vi "Wait On Timer Example 2.vi"() -> ()   [LabVIEW 2011]
panel:
  out "Exit":bool
  in  "Stop":bool
  out "Waveform Chart":dbl[](graph)
  in  "Time between chart updates (sec)":dbl=0.5 format="%.3f"
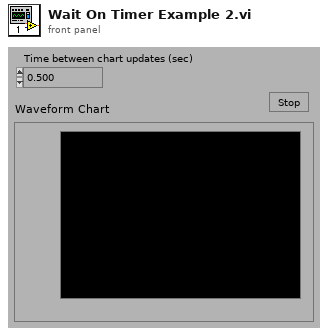
[diagram p1: front panel]
types:
  T1 = typedef "Timer Refnum.ctl" = refnum<k1>
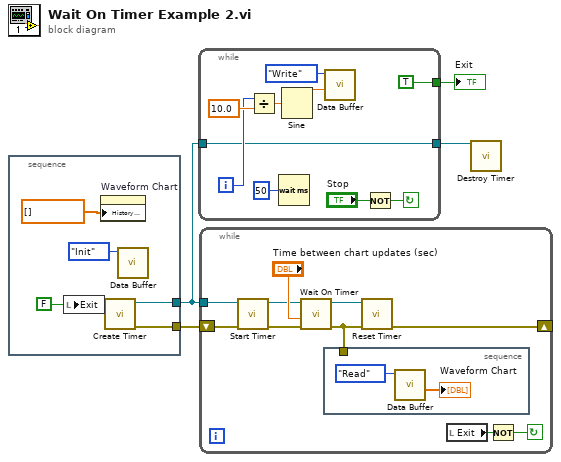
[diagram p0: block diagram]
diagram:
  n1 = stacked-sequence {
    tunnel: [w9] -> w3
    tunnel: [w8] -> w4
    frame #0 {
      n2 = local write "Exit"(FALSE ("Exit")) -> ()
      n3 = property on="Waveform Chart" class="WFChart (strict)"("History Data"=dbl[] [] ("Write Attribute")) -> ()  [unwired: 2 in, 2 out]
      n4 = call "Create Timer.vi"() -> ("error out"=w8:errorcluster, "timer"=w9:T1)  [unwired: 5 in, 1 out]
      n5 = call "Data Buffer.vi"("task"=enum16{"Init", "Write", "Read"}."Init") -> ()  [unwired: 6 in, 1 out]
    }
  }
  n6 = while {
    tunnel: [TRUE ("Stop")] -> w1
    tunnel: [w11] -> w2
    tunnel: w3 -> [w11]
    i -> [w18]
    stop <- w13 continue-if-true
    n7 = Divide(x=w18, y=10.0) -> (x/y=w17:dbl)
    n8 = Wait (ms)(milliseconds to wait=u32 50) -> ()  [unwired: 1 out]
    n9 = Sine(x=w17) -> (sin(x)=w15:dbl)
    n10 = call "Data Buffer.vi"("Datum in"=w15, "task"=enum16{"Init", "Write", "Read"}."Write") -> ()  [unwired: 5 in, 1 out]
    n11 = Not(x="Stop") -> (.not. x?=w13:bool)
  }
  "Exit" <- w1
  n12 = while {
    shift-left: w4 -> [w28]
    shift-right: [w23] -> _
    tunnel: w3 -> [w25]
    stop <- w20 continue-if-true
    n13 = call "Start Timer.vi"("error in (no error)"=w28, "timer"=w25) -> ("error out"=w27:errorcluster, "timer out"=w26:T1)  [unwired: 8 in]
    n14 = call "Wait On Timer.vi"("error in (no error)"=w27, "timer value to wait for in seconds"="Time between chart updates (sec)", "timer"=w26) -> ("error out"=w22:errorcluster, "timer out"=w24:T1)  [unwired: 2 in, 1 out]
    n15 = stacked-sequence {
      tunnel: w22 -> [_]
      frame #0 {
        n16 = call "Data Buffer.vi"("task"=enum16{"Init", "Write", "Read"}."Read") -> ("Data out"=→"Waveform Chart":dbl[])  [unwired: 6 in]
      }
    }
    n17 = call "Reset Timer.vi"("error in (no error)"=w22, "timer"=w24) -> ("error out"=w23:errorcluster)  [unwired: 8 in, 1 out]
    n18 = local read "Exit"() -> (w21:bool)
    n19 = Not(x=w21) -> (.not. x?=w20:bool)
  }
  n20 = call "Destroy Timer.vi"("timer"=w2) -> ()  [unwired: 5 in, 2 out]
